vi "Signal Reload Config Event.vi"   [LabVIEW 2013]
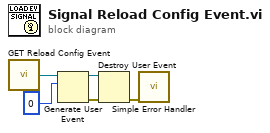
[diagram p0: block diagram]
diagram:
  n1 = call "GET Reload Config Event.vi"() -> ("Reload Config Event"=w1:refnum<user-event>)
  n2 = Generate User Event(user event=w1, event data cluster=0 ("event data")) -> (user event out=w3:refnum<user-event>, error out=w4:errorcluster)  [unwired: 2 in]
  n3 = Destroy User Event(user event=w3, error in=w4) -> (error out=w5:errorcluster)
  n4 = call <vilib>:"Simple Error Handler.vi"("error in (no error)"=w5) -> ()  [unwired: 4 in, 5 out]
